vi "sc5511a_spf_select_devices.vi"(5 "error in (no error)":errorcluster) -> (14 "Selected Resource":string, 19 "error out":errorcluster)   [LabVIEW 2010]
panel:
  in  "Cancel Button 2":bool
  in  "OK Button 2":bool
  out "source":string="No SC800  Found."
  in  "Resource Name":u16(ring)
  # "Please select a device from the pull-down menu:"
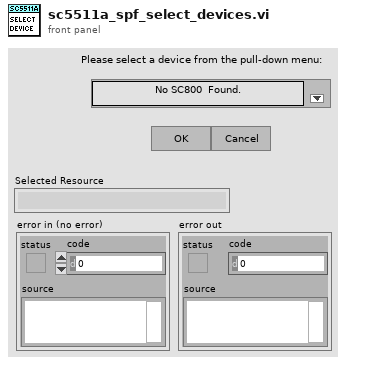
[diagram p1: front panel]
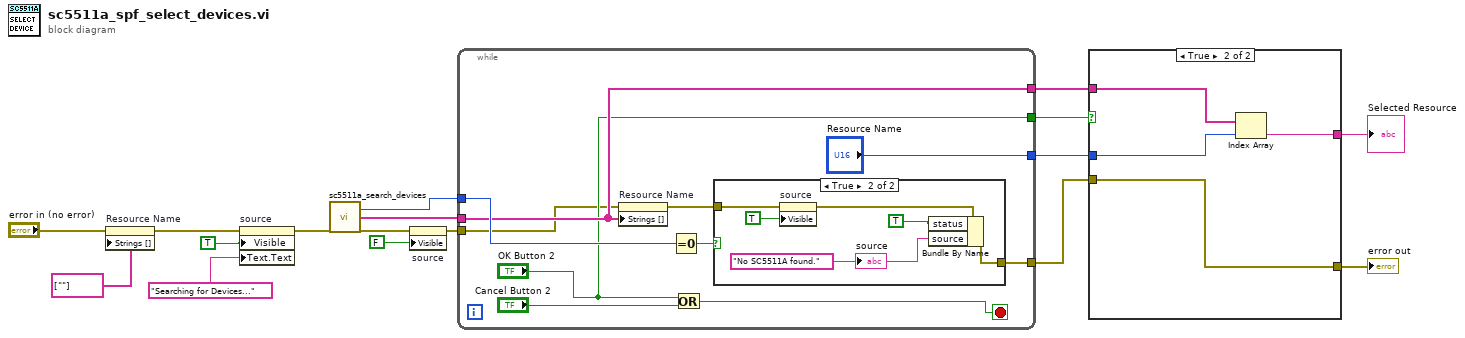
[diagram p0: block diagram]
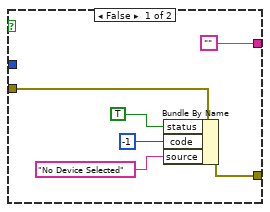
[diagram p2: hidden frame]
diagram:
  n1 = property on="Resource Name" class="Ring (strict)"(error in="error in (no error)", "Strings []"=string[] [""]) -> (error out=w9:errorcluster)  [unwired: 1 in, 1 out]
  n2 = property on="source" class="Str"(error in=w9, "Visible"=TRUE, "Text.Text"="Searching for Devices...") -> (error out=w7:errorcluster)  [unwired: 1 in, 1 out]
  n3 = call "sc5511a_search_devices.vi"("error in (no error)"=w7) -> ("Number of Devices"=w6:i32, "Device SN"=w5:string[], "error out"=w3:errorcluster)  [unwired: 16 in]
  n4 = property on="source" class="Str"(error in=w3, "Visible"=FALSE) -> (error out=w2:errorcluster)  [unwired: 1 in, 1 out]
  n5 = while {
    tunnel: ["Resource Name"] -> w16
    tunnel: [w21] -> w17
    tunnel: ["OK Button 2"] -> w15
    tunnel: w2 -> [w18]
    tunnel: [w24] -> w11
    tunnel: w6 -> [w22]
    tunnel: w5 -> [w21]
    stop <- w23 stop-if-true
    n6 = property on="Resource Name" class="Ring (strict)"(error in=w18, "Strings []"=w21) -> (error out=w25:errorcluster)  [unwired: 1 in, 1 out]
    n7 = Equal To 0?(x=w22) -> (x = 0?=w26:bool)
    n8 = Or(x="OK Button 2", y="Cancel Button 2") -> (x .or. y?=w23:bool)
    n9 = case shown="True" w26 {
      tunnel: w25 -> [w28 w31]
      tunnel: [w28 w34] -> w24
      frame False {
      }
      frame True {
        w29 = "No SC5511A found." ("source")
        n10 = property on="source" class="Str"(error in=w31, "Visible"=TRUE) -> (error out=w32:errorcluster)  [unwired: 1 in, 1 out]
        n11 = Bundle By Name(cluster=w32, "status"=TRUE, "source"=w29) -> (w34:errorcluster)
        "source" <- w29
      }
    }
  }
  n12 = case shown="True" w15 {
    tunnel: w17 -> [_ w44]
    tunnel: w16 -> [_ w43]
    tunnel: ["" w42] -> w14
    tunnel: w11 -> [w39 w41]
    tunnel: [w37 w41] -> w10
    frame False {
      n13 = Bundle By Name(cluster=w39, "status"=TRUE, "code"=-1, "source"="No Device Selected") -> (w37:errorcluster)
    }
    frame True {
      n14 = Index Array(array=w44, index=w43) -> (element=w42:string)
    }
  }
  "Selected Resource" <- w14
  "error out" <- w10
